vi "PI Connect Sequence.vi"(8 "error in (no error)":errorcluster) -> (0 "error out":errorcluster, 2 "PreLaunchStagePos":T1={"Position (SET)"={"XaxesSET"=0.0, "YaxesSET"=0.0}, "Position (ACT)"={"PosXACT"=0.0087, "PosYACT"=0.0087}} caption="output cluster" {"Position (ACT)"."PosYACT" min=0.0 max=220.0 step=0.1 format="%.2f"; "Position (ACT)"."PosXACT" min=0.0 max=220.0 step=0.1 format="%.2f"; "Position (SET)"."YaxesSET" min=0.0 max=220.0 step=0.1 scale=0.0..220.0; "Position (SET)"."XaxesSET" min=0.0 max=220.0 step=0.1 scale=0.0..220.0}, 3 "Boolean":bool)   [LabVIEW 2020]
uses:
  PI Settings.ctl
  PI Settings Global.vi
  Low Level/Communication.llb/Global1.vi
  Low Level/Communication.llb/Available DLL interfaces.ctl
  Low Level/Communication.llb/Available DLLs.ctl
  PI Position.ctl
panel:
  out "Conn. Axes":string[](array[string])
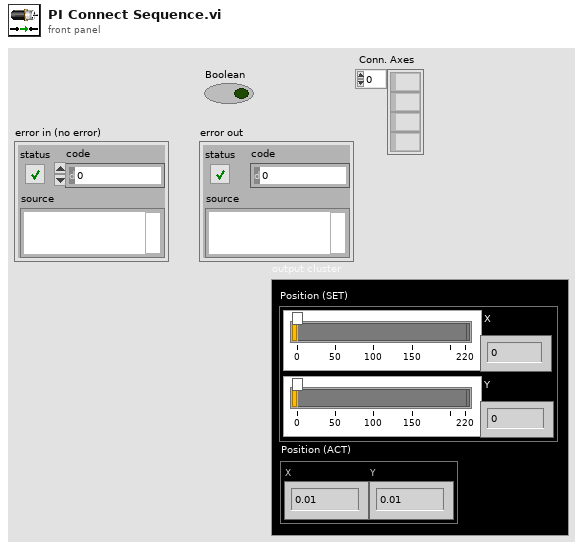
[diagram p1: front panel]
types:
  T1 = typedef "PI Position.ctl" = cluster{"Position (SET)":cluster{"XaxesSET":dbl, "YaxesSET":dbl}, "Position (ACT)":cluster{"PosXACT":dbl, "PosYACT":dbl}}
  T2 = typedef "PI Settings.ctl" = cluster{"System number":i32, "Commanded axes":string[], "Controller error":bool, "Error":errorcluster}
  T3 = typedef "Available DLLs.ctl" = u16
  T4 = typedef "Available DLL interfaces.ctl" = u16
  T5 = cluster{"DLL for Device":T3, "DLL Interface":T4, "Parameter":string}[]
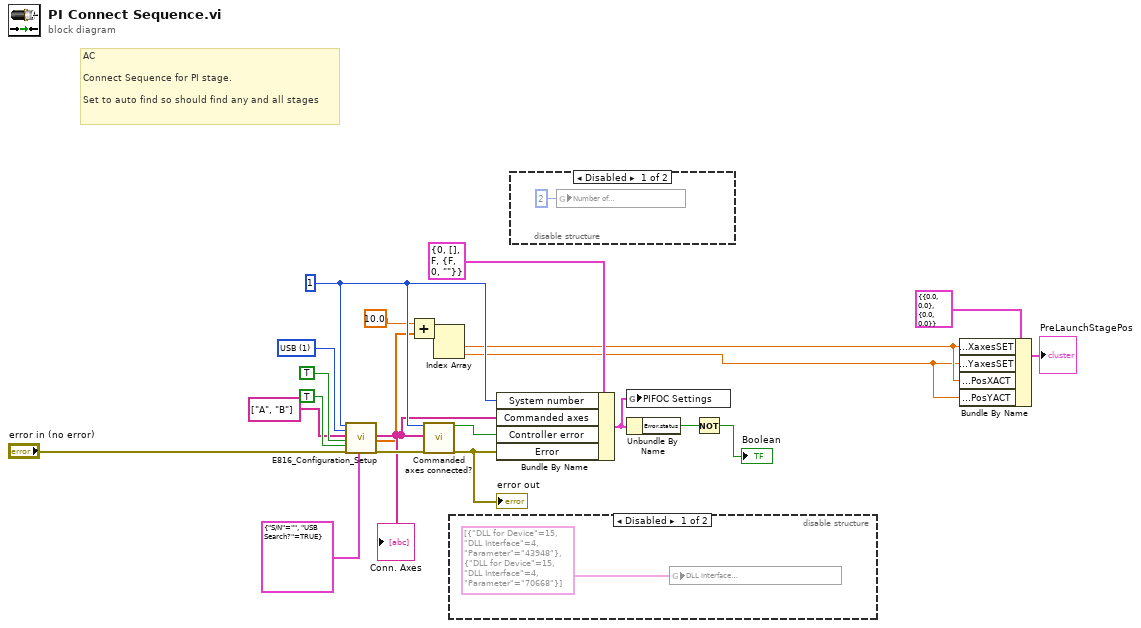
[diagram p0: block diagram]
diagram:
  w14 = u16 1 items=["RS232", "USB"] ("Interface")
  w12 = 1 ("System no.")
  # "AC\n\nConnect Sequence for PI stage.\n\nSet to auto find so should find any and all stages"
  n1 = call "E816_Configuration_Setup.vi"("System no."=w12, "Interface"=w14, "Axes to move"=string[] ["A", "B"], "All axes?"=TRUE, "Change servo \nstatus to ON?"=TRUE ("Use dialog to define\nconnected stages?"), "error in"="error in (no error)", "USB settings"=cluster{"S/N":string, "USB Search?":bool} {"S/N"="", "USB Search?"=TRUE}) -> ("Conn. Axes"=w10:string[], "Position"=w6:dbl[], "error out"=w13:errorcluster)  [unwired: 8 in, 2 out]
  "Conn. Axes" <- w10
  n2 = Add(x=10.0, y=w6) -> (x+y=w2:dbl[])
  n3 = call "Commanded axes connected?.vi"("System no."=w12, "Commanded axes"=w10, "error in"=w13) -> ("Controller error"=w11:bool, "error out"=w19:errorcluster)  [unwired: 15 in]
  "error out" <- w19
  n4 = Index Array(array=w2) -> (element #1=w4:dbl, element #2=w3:dbl)  [unwired: 2 in]
  n5 = disable-structure shown="Disabled" {
    frame Disabled {
      n6 = global write "Global1.vi" "DLL Interface\nConfiguration"(T5 [{"DLL for Device"=15, "DLL Interface"=4, "Parameter"="43948"}, {"DLL for Device"=15, "DLL Interface"=4, "Parameter"="70668"}] ("DLL Interface\nConfiguration")) -> ()
    }
    frame Enabled {
    }
  }
  n7 = Bundle By Name(cluster=T2 {"System number"=0, "Commanded axes"=[], "Controller error"=FALSE, "Error"={"status"=FALSE, "code"=0, "source"=""}} ("PIFOC Position 2"), "System number"=w12, "Commanded axes"=w10, "Controller error"=w11, "Error"=w19) -> (w22:T2)
  n8 = disable-structure shown="Disabled" {
    frame Disabled {
      n9 = global write "Global1.vi" "Number of\nsystems"(2 ("Number of\nsystems")) -> ()
    }
    frame Enabled {
    }
  }
  n10 = global write "PI Settings Global.vi" "PIFOC Settings"(w22) -> ()
  n11 = Unbundle By Name(w22) -> ("Error.status"=w16:bool)
  n12 = Not(x=w16) -> (.not. x?=→"Boolean":bool)
  n13 = Bundle By Name(cluster=T1 {"Position (SET)"={"XaxesSET"=0.0, "YaxesSET"=0.0}, "Position (ACT)"={"PosXACT"=0.0, "PosYACT"=0.0}} ("Stage Position"), "Position (SET).XaxesSET"=w4, "Position (SET).YaxesSET"=w3, "Position (ACT).PosXACT"=w4, "Position (ACT).PosYACT"=w3) -> (→"PreLaunchStagePos":T1)
